vi "Save Configuration.vi"(8 "error in (no error)":errorcluster, 11 "Measurement Setup UI in":refnum<class "Measurement Setup UI.lvclass">) -> (0 "error out":errorcluster, 3 "Measurement Setup UI out":refnum<class "Measurement Setup UI.lvclass">)   [LabVIEW 2017, in "Measurement Setup Controller.lvlib" / "Measurement Setup UI.lvclass"]
uses:
  Measurement Setup UI.lvclass
  C:/Program Files (x86)/National Instruments/LabVIEW 2017/user.lib/Common Components/Msmt UI/Measurement UI.lvclass
  C:/Program Files (x86)/National Instruments/LabVIEW 2017/vi.lib/ActorFramework/Actor/Actor.lvclass
  Measurement Data/Measurement Data.lvclass
  Measurement Data/Measurement Data.lvclass/Measurement Data.ctl
  <vilib>/ActorFramework/Actor/Actor.lvclass/Actor.ctl
  Measurement Setup Messages/Store Measuement Config Msg/Store Measuement Config Msg.lvclass/Store Measuement Config Msg.ctl
  <vilib>/ActorFramework/Message Enqueuer/Message Enqueuer.lvclass/Message Enqueuer.ctl
  <vilib>/ActorFramework/Message Enqueuer/Enqueue.vi
  Measurement Setup Messages/Store Measuement Config Msg/Store Measuement Config Msg.lvclass
  C:/Program Files (x86)/National Instruments/LabVIEW 2017/vi.lib/ActorFramework/Message/Message.lvclass
  <vilib>/ActorFramework/Message Priority Queue/Priority Enqueue.vi
  <userlib>/Common Components/Msmt UI/Measurement UI.lvclass
  <vilib>/ActorFramework/Actor/Actor.lvclass
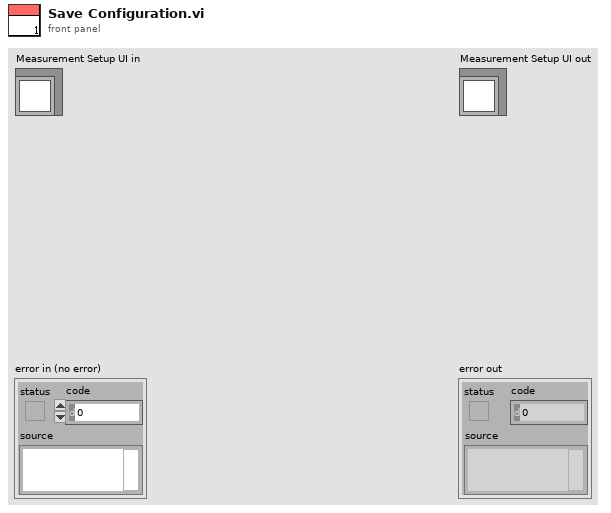
[diagram p1: front panel]
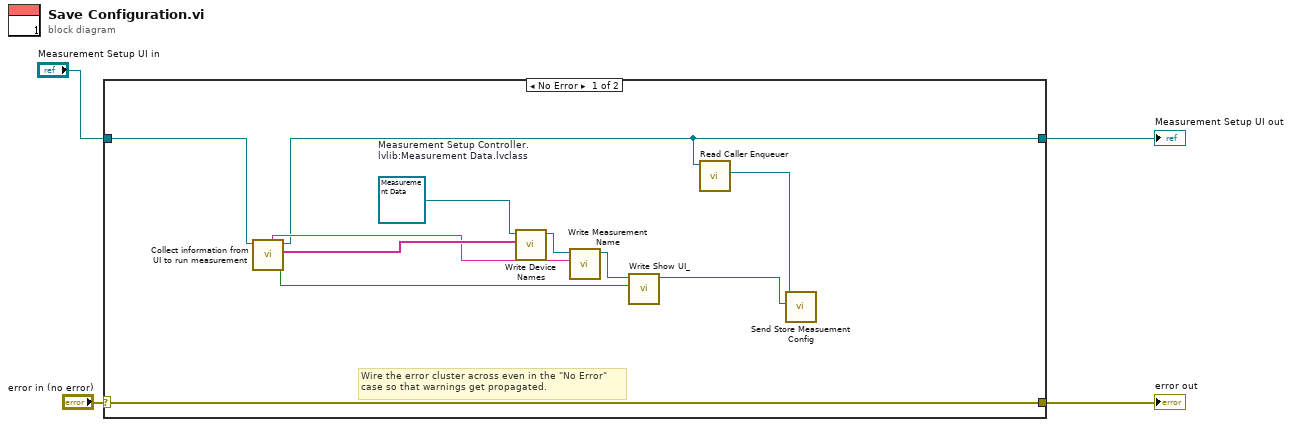
[diagram p0: block diagram]
diagram:
  n1 = case shown="No Error" "error in (no error)" {
    selector: "error in (no error)" -> [w15 w17]
    tunnel: [w15 w17] -> w3
    tunnel: [w5 w16] -> w1
    tunnel: "Measurement Setup UI in" -> [w14 w16]
    frame No Error {
      w13 = refnum<class "Measurement Data.lvclass"> refnum  # Measurement Setup Controller.lvlib:Measurement Data.lvclass
      # "Wire the error cluster across even in the \"No Error\"\ncase so that warnings get propagated."
      n2 = call <userlib>:"Collect information from UI to run measurement.vi"("Measurement UI in"=w14) -> ("Show UI?"=w10:bool, "Device Names"=w12:string[], "Measurement UI out"=w5:refnum<class "Measurement Setup UI.lvclass">, "Measurement Name"=w11:string)  [unwired: 3 in, 4 out]
      n3 = call "Write Device Names.vi"("Device Names"=w12, "Measurement Data in"=w13) -> ("Measurement Data out"=w9:refnum<class "Measurement Data.lvclass">)  [unwired: 8 in, 1 out]
      n4 = call "Write Measurement Name.vi"("Measurement Name"=w11, "Measurement Data in"=w9) -> ("Measurement Data out"=w8:refnum<class "Measurement Data.lvclass">)  [unwired: 8 in, 1 out]
      n5 = call "Write Show UI_.vi"("Show UI?"=w10, "Measurement Data in"=w8) -> ("Measurement Data out"=w7:refnum<class "Measurement Data.lvclass">)  [unwired: 8 in, 1 out]
      n6 = call <vilib>:"Read Caller Enqueuer.vi"("Actor"=w5) -> ("Caller Enqueuer"=w6:refnum<class "Message Enqueuer.lvclass">)  [unwired: 10 in]
      n7 = call "Send Store Measuement Config.vi"("Measurement Setup Controller.lvlib:Measurement Data.lvclass"=w7, "Message Enqueuer"=w6) -> ()  [unwired: 8 in, 2 out]
    }
    frame Error {
    }
  }
  "error out" <- w3
  "Measurement Setup UI out" <- w1
